vi "Populate Yokogawa Settings.vi"(4 "Sample Rate":string[](array[string]), 5 "Power  in":T2={"Yokogawa"={"WT210"={"Sample Rate (1: 0.25s)"=1, "A Range (12: 20A)"=11, "V Range (6: 600V)"=4, "Power VISA Yokogawa WT210"=""}, "WT500"={"Power VISA Yokogawa WT500"="", "V Range (8: 1000V)"=6, "I Range (7: 40A)"=7, "Update Rate (3: 500ms)"=2}}, "Aplus"={"Aplus IP Address"="192.168.1.101", "Remote Port"=502, "Instrument"="APLUS", "Instr Driver Revision"="1.03.0053"}, "Power Limits"={"Crest Factor"={"Upper Limit"=1.49, "Lower Limit"=1.34}, "Harmonic Content"={"Uthd"=2.0}, "Voltage"={"% Error"=2.0}, "Stability"={"<1 Watt "={"Wattage"=1.0, "Slope (mW/H)"=10.0}, ">1 Watt"={"1%Power/Hour"=1.0}}}, "Nominal Voltage"=120, "Time Limit (s)"=10800.0, "Power Variation Limit (%)"=50.0, "Power Supply"={"Chroma 61605"="CHROMA", "Use Chroma?"=FALSE}} {"Yokogawa"."WT500"."Update Rate (3: 500ms)" items=["-", "100ms", "200ms", "500ms", "1s", "2s", "5s"]; "Yokogawa"."WT500"."I Range (7: 40A)" items=["AUTO", "500 mA", "1 A", "2 A", "5 A", "10 A", "20 A", "40 A", "S-AUTO", "50 mV", "100 mV", "200 mV", "500 mV", "1 V", "2 V", "5 V", "10 V", "250 mA", "500 mA", "1 A", "2.5 A", "5 A", "10 A", "20 A", "25 mV", "50 mV", "100 mV", "250 mV", "500 mV", "1 V", "2.5 V", "5 V"]; "Yokogawa"."WT500"."V Range (8: 1000V)" items=["AUTO", "15", "30", "60", "100", "150", "300", "600", "1000", "7.5", "15", "30", "50", "75", "150", "300", "500"]; "Yokogawa"."WT210"."V Range (6: 600V)" items=["Auto", "15V", "30V", "60V", "150V", "300V", "600V"]; "Yokogawa"."WT210"."A Range (12: 20A)" items=["Auto", "5mA", "10mA", "20mA", "50mA", "100mA", "200mA", "0.5A", "1A", "2A", "5A", "10A", "20A", "50mV", "100mV", "200mV", "2.5V", "5V", "10V"]; "Yokogawa"."WT210"."Sample Rate (1: 0.25s)" items=["0.1s", "0.25s", "0.5s", "1s", "2s", "5s"]}, 6 "A Range":string[](array[string]), 7 "Input Array":string[][](array[string]), 8 "error in (no error)":errorcluster, 9 "V Range":string[](array[string]), 11 "Power Analyzer":T1=enum."APLUS") -> (0 "error out":errorcluster, 3 "Power  out":T2={"Yokogawa"={"WT210"={"Sample Rate (1: 0.25s)"=1, "A Range (12: 20A)"=11, "V Range (6: 600V)"=4, "Power VISA Yokogawa WT210"=""}, "WT500"={"Power VISA Yokogawa WT500"="", "V Range (8: 1000V)"=6, "I Range (7: 40A)"=7, "Update Rate (3: 500ms)"=2}}, "Aplus"={"Aplus IP Address"="192.168.1.101", "Remote Port"=502, "Instrument"="APLUS", "Instr Driver Revision"="1.03.0053"}, "Power Limits"={"Crest Factor"={"Upper Limit"=1.49, "Lower Limit"=1.34}, "Harmonic Content"={"Uthd"=2.0}, "Voltage"={"% Error"=2.0}, "Stability"={"<1 Watt "={"Wattage"=1.0, "Slope (mW/H)"=10.0}, ">1 Watt"={"1%Power/Hour"=1.0}}}, "Nominal Voltage"=120, "Time Limit (s)"=10800.0, "Power Variation Limit (%)"=50.0, "Power Supply"={"Chroma 61605"="CHROMA", "Use Chroma?"=FALSE}} {"Yokogawa"."WT500"."Update Rate (3: 500ms)" items=["-", "100ms", "200ms", "500ms", "1s", "2s", "5s"]; "Yokogawa"."WT500"."I Range (7: 40A)" items=["AUTO", "500 mA", "1 A", "2 A", "5 A", "10 A", "20 A", "40 A", "S-AUTO", "50 mV", "100 mV", "200 mV", "500 mV", "1 V", "2 V", "5 V", "10 V", "250 mA", "500 mA", "1 A", "2.5 A", "5 A", "10 A", "20 A", "25 mV", "50 mV", "100 mV", "250 mV", "500 mV", "1 V", "2.5 V", "5 V"]; "Yokogawa"."WT500"."V Range (8: 1000V)" items=["AUTO", "15", "30", "60", "100", "150", "300", "600", "1000", "7.5", "15", "30", "50", "75", "150", "300", "500"]; "Yokogawa"."WT210"."V Range (6: 600V)" items=["Auto", "15V", "30V", "60V", "150V", "300V", "600V"]; "Yokogawa"."WT210"."A Range (12: 20A)" items=["Auto", "5mA", "10mA", "20mA", "50mA", "100mA", "200mA", "0.5A", "1A", "2A", "5A", "10A", "20A", "50mV", "100mV", "200mV", "2.5V", "5V", "10V"]; "Yokogawa"."WT210"."Sample Rate (1: 0.25s)" items=["0.1s", "0.25s", "0.5s", "1s", "2s", "5s"]})   [LabVIEW 2016]
uses:
  Type Definitions/UTILITY Power Inputs Control.ctl
  Type Definitions/UTILITY Power Analyzer.ctl
  <vilib>/Instr/_visa.llb/VISA Find Search Mode.ctl
  <vilib>/Utility/error.llb/whitespace.ctl
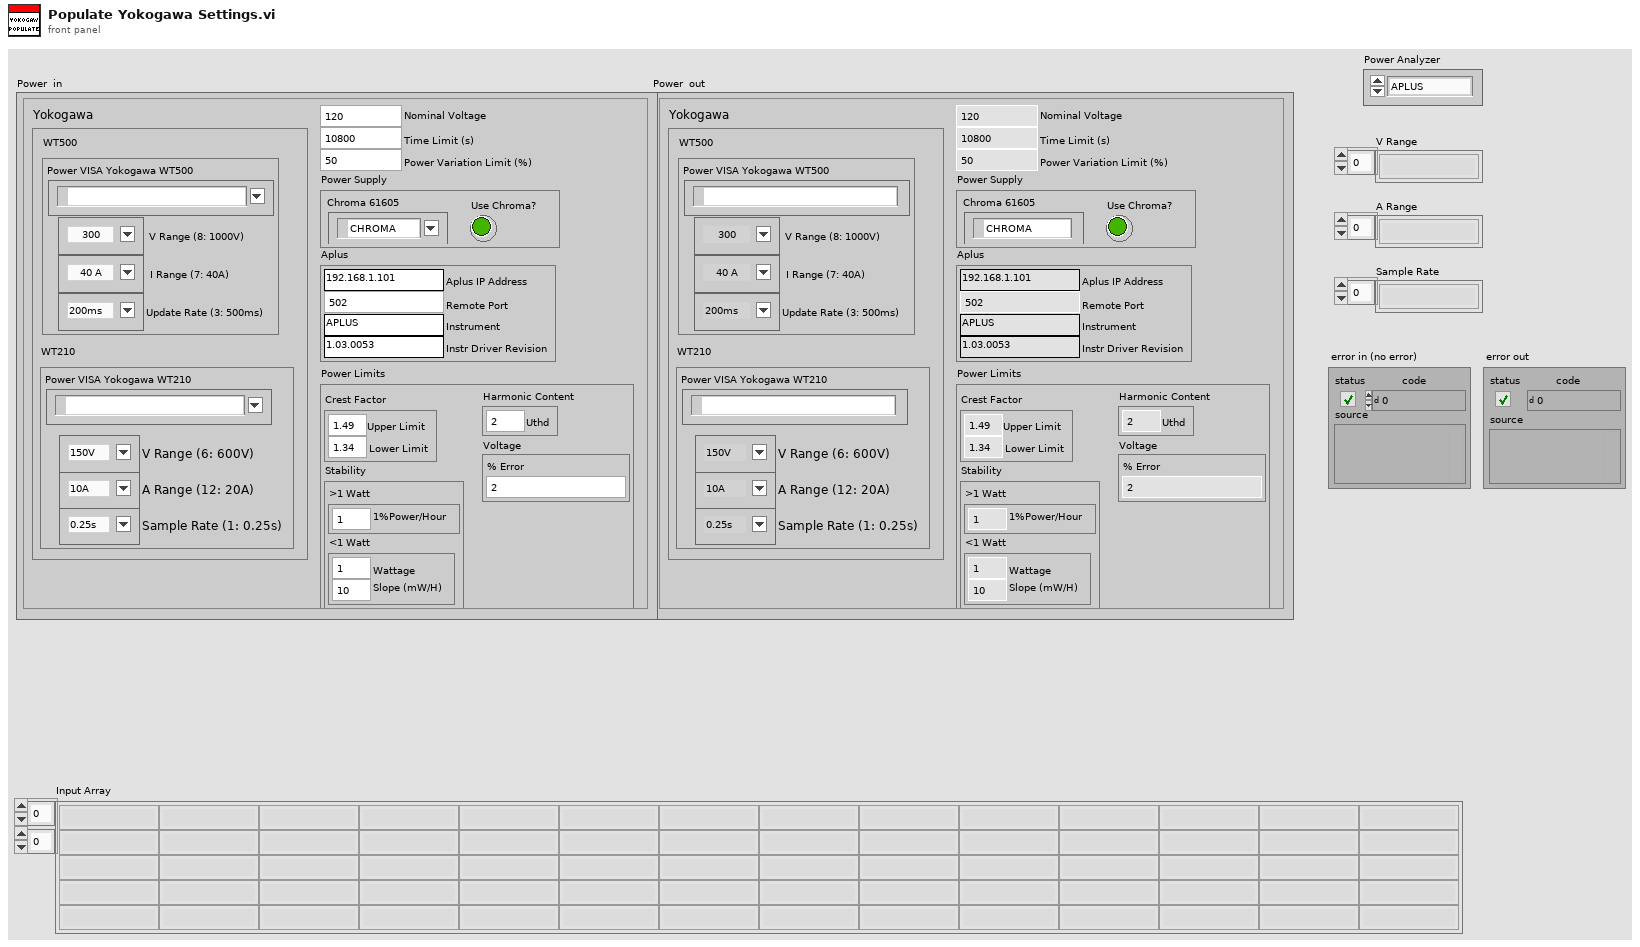
[diagram p1: front panel]
types:
  T1 = typedef "UTILITY Power Analyzer.ctl" = enum16{"", "APLUS", "WT210", "WT500", "WT300", "OSI", "Debug", "WT230"}
  T2 = typedef "UTILITY Power Inputs Control.ctl" = cluster{"Yokogawa":cluster{"WT210":cluster{"Sample Rate (1: 0.25s)":i32, "A Range (12: 20A)":i32, "V Range (6: 600V)":i32, "Power VISA Yokogawa WT210":refnum<visa-resource-name>}, "WT500":cluster{"Power VISA Yokogawa WT500":refnum<visa-resource-name>, "V Range (8: 1000V)":i32, "I Range (7: 40A)":i32, "Update Rate (3: 500ms)":i32}}, "Aplus":cluster{"Aplus IP Address":string, "Remote Port":i32, "Instrument":string, "Instr Driver Revision":string}, "Power Limits":cluster{"Crest Factor":cluster{"Upper Limit":dbl, "Lower Limit":dbl}, "Harmonic Content":cluster{"Uthd":dbl}, "Voltage":cluster{"% Error":dbl}, "Stability":cluster{"<1 Watt ":cluster{"Wattage":dbl, "Slope (mW/H)":dbl}, ">1 Watt":cluster{"1%Power/Hour":dbl}}}, "Nominal Voltage":i32, "Time Limit (s)":dbl, "Power Variation Limit (%)":dbl, "Power Supply":cluster{"Chroma 61605":refnum<visa-resource-name>, "Use Chroma?":bool}}
  T3 = typedef "VISA Find Search Mode.ctl" = u32
  T4 = typedef "whitespace.ctl" = u16
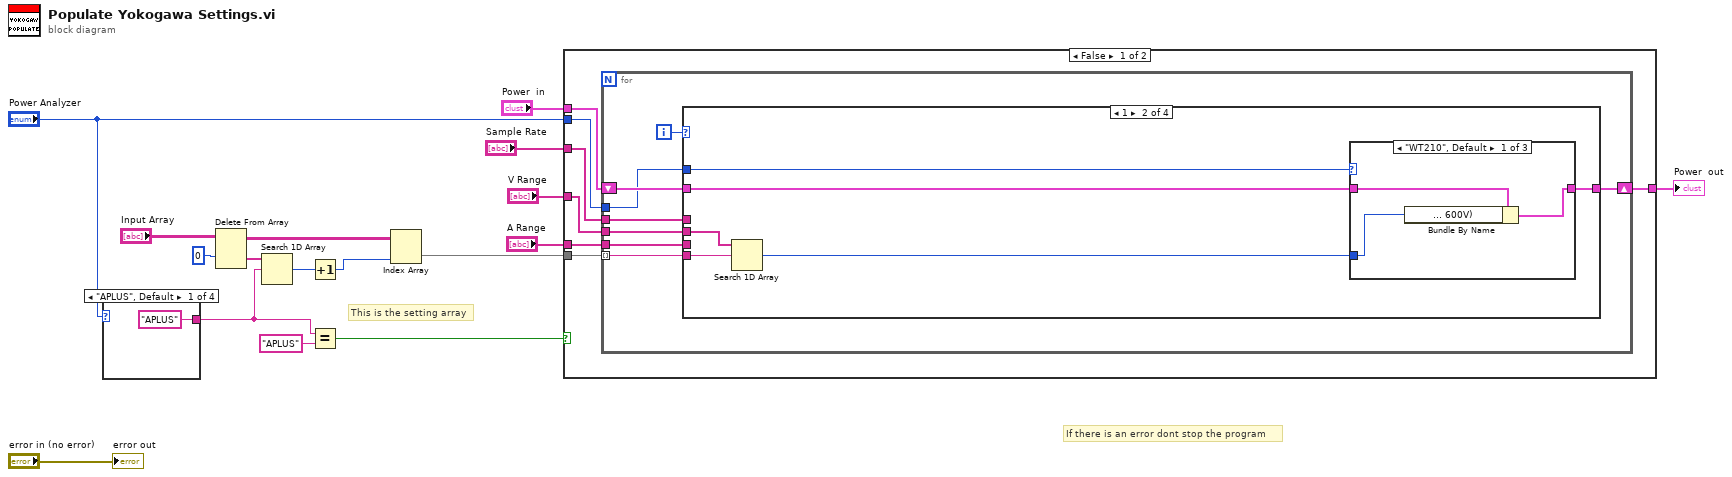
[diagram p0: block diagram]
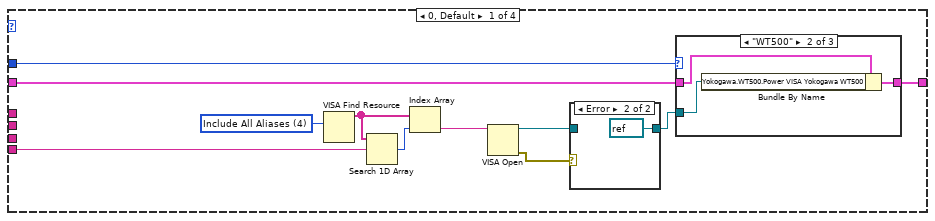
[diagram p2: hidden frame]
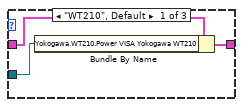
[diagram p4: hidden frame]
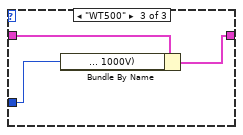
[diagram p7: hidden frame]
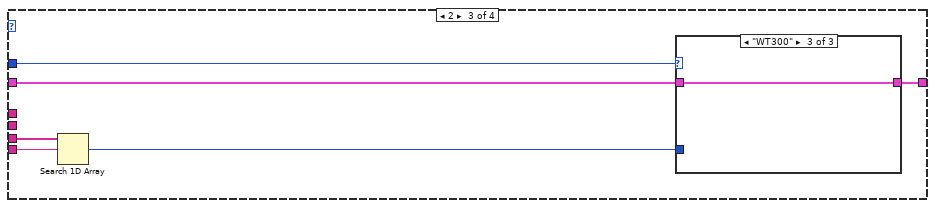
[diagram p8: hidden frame]
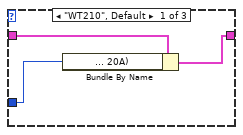
[diagram p9: hidden frame]
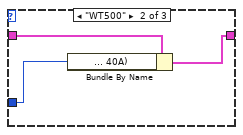
[diagram p10: hidden frame]
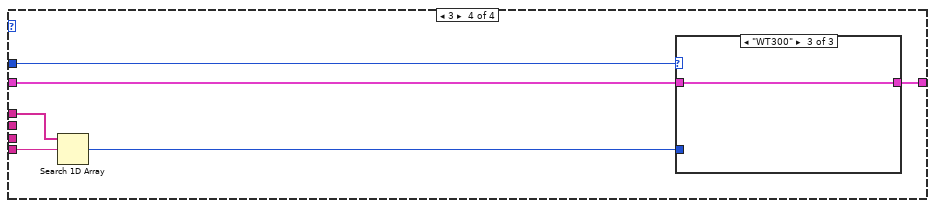
[diagram p11: hidden frame]
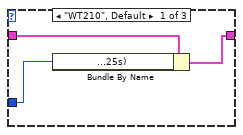
[diagram p12: hidden frame]
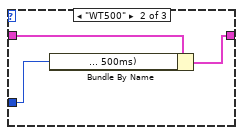
[diagram p13: hidden frame]
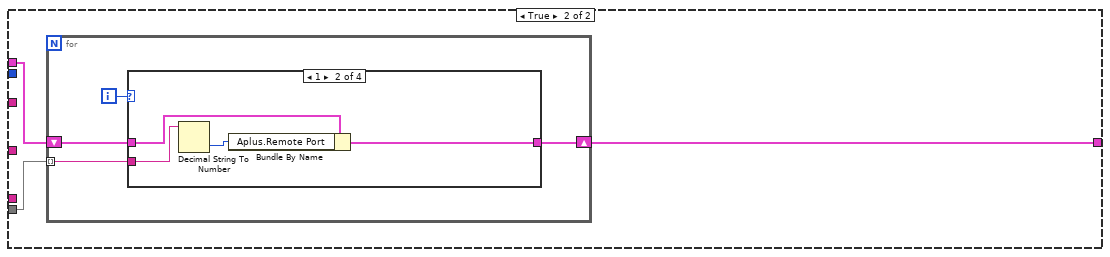
[diagram p14: hidden frame]
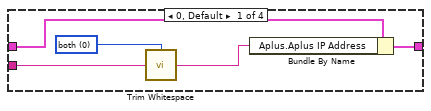
[diagram p15: hidden frame]
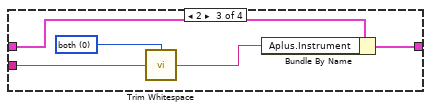
[diagram p16: hidden frame]
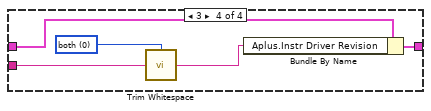
[diagram p17: hidden frame]
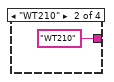
[diagram p18: hidden frame]
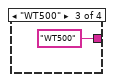
[diagram p19: hidden frame]
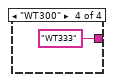
[diagram p20: hidden frame]
diagram:
  # "If there is an error dont stop the program"
  # "This is the setting array"
  n1 = case shown="\"APLUS\", Default" "Power Analyzer" {
    tunnel: ["APLUS" "WT210" "WT500" "WT333"] -> w2
    frame "APLUS", Default {
    }
    frame "WT210" {
    }
    frame "WT500" {
    }
    frame "WT300" {
    }
  }
  n2 = Delete From Array(array="Input Array", index (row)=0) -> (deleted portion=w7:string[], array with subset deleted=w8:string[][])  [unwired: 2 in]
  n3 = Search 1D Array(1D array=w7, element=w2) -> (index of element=w5:i32)  [unwired: 1 in]
  n4 = Increment(x=w5) -> (x+1=w12:i32)
  n5 = Equal?(x=w2, y="APLUS") -> (x = y?=w4:bool)
  n6 = Index Array(array=w8, index (col)=w12) -> (element=w11:string[])  [unwired: 1 in]
  n7 = case shown="False" w4 {
    tunnel: "Sample Rate" -> [w28 _]
    tunnel: "A Range" -> [w27 _]
    tunnel: "V Range" -> [w26 _]
    tunnel: [w25 w96] -> w14
    tunnel: "Power  in" -> [w24 w97]
    tunnel: w11 -> [w23 w98]
    tunnel: "Power Analyzer" -> [w22 _]
    frame False {
      n8 = for {
        tunnel: w23 -> [w34] mode=indexing
        shift-right: [w33] -> w25
        shift-left: w24 -> [w35]
        tunnel: w22 -> [w32]
        tunnel: w26 -> [w31]
        tunnel: w27 -> [w30]
        tunnel: w28 -> [w29]
        i -> [w36]
        n9 = case shown="1" w36 {
          tunnel: w35 -> [w47 w62 w75 w88]
          tunnel: [w46 w61 w74 w87] -> w33
          tunnel: w34 -> [w41 w60 w73 w86]
          tunnel: w32 -> [w40 w57 w70 w83]
          tunnel: w31 -> [_ w58 _ _]
          tunnel: w30 -> [_ _ w71 _]
          tunnel: w29 -> [_ _ _ w84]
          frame 0, Default {
            w45 = T3 4 items=["Canonical Names Only"=0, "Aliases Only"=2, "Include Matching Aliases"=3, "Include All Aliases"=4] ("Search Mode")
            n10 = VISA Find Resource(10:w45) -> (3:w43:string[])  [unwired: 2 in, 2 out]
            n11 = Search 1D Array(1D array=w43, element=w41) -> (index of element=w44:i32)  [unwired: 1 in]
            n12 = Index Array(array=w43, index=w44) -> (element=w42:string)
            n13 = VISA Open(VISA resource name=w42) -> (VISA resource name=w38:refnum<visa-resource-name>, error out=w39:errorcluster)  [unwired: 4 in]
            n14 = case shown="Error" w39 {
              tunnel: w38 -> [w48 _]
              tunnel: [w48 refnum<visa-resource-name> refnum ("VISA resource name")] -> w37
              frame No Error {
              }
              frame Error {
              }
            }
            n15 = case shown="\"WT500\"" w40 {
              tunnel: w47 -> [w52 w55 w56]
              tunnel: [w51 w54 w56] -> w46
              tunnel: w37 -> [w50 w53 _]
              frame "WT210", Default {
                n16 = Bundle By Name(cluster=w52, "Yokogawa.WT210.Power VISA Yokogawa WT210"=w50) -> (w51:T2)
              }
              frame "WT500" {
                n17 = Bundle By Name(cluster=w55, "Yokogawa.WT500.Power VISA Yokogawa WT500"=w53) -> (w54:T2)
              }
              frame "WT300" {
              }
            }
          }
          frame 1 {
            n18 = Search 1D Array(1D array=w58, element=w60) -> (index of element=w59:i32)  [unwired: 1 in]
            n19 = case shown="\"WT210\", Default" w57 {
              tunnel: w62 -> [w65 w66 w69]
              tunnel: [w64 w66 w68] -> w61
              tunnel: w59 -> [w63 _ w67]
              frame "WT210", Default {
                n20 = Bundle By Name(cluster=w65, "Yokogawa.WT210.V Range (6: 600V)"=w63) -> (w64:T2)
              }
              frame "WT300" {
              }
              frame "WT500" {
                n21 = Bundle By Name(cluster=w69, "Yokogawa.WT500.V Range (8: 1000V)"=w67) -> (w68:T2)
              }
            }
          }
          frame 2 {
            n22 = Search 1D Array(1D array=w71, element=w73) -> (index of element=w72:i32)  [unwired: 1 in]
            n23 = case shown="\"WT300\"" w70 {
              tunnel: w75 -> [w77 w81 w82]
              tunnel: [w78 w80 w82] -> w74
              tunnel: w72 -> [w76 w79 _]
              frame "WT210", Default {
                n24 = Bundle By Name(cluster=w77, "Yokogawa.WT210.A Range (12: 20A)"=w76) -> (w78:T2)
              }
              frame "WT500" {
                n25 = Bundle By Name(cluster=w81, "Yokogawa.WT500.I Range (7: 40A)"=w79) -> (w80:T2)
              }
              frame "WT300" {
              }
            }
          }
          frame 3 {
            n26 = Search 1D Array(1D array=w84, element=w86) -> (index of element=w85:i32)  [unwired: 1 in]
            n27 = case shown="\"WT300\"" w83 {
              tunnel: w88 -> [w89 w94 w95]
              tunnel: [w90 w93 w95] -> w87
              tunnel: w85 -> [w91 w92 _]
              frame "WT210", Default {
                n28 = Bundle By Name(cluster=w89, "Yokogawa.WT210.Sample Rate (1: 0.25s)"=w91) -> (w90:T2)
              }
              frame "WT500" {
                n29 = Bundle By Name(cluster=w94, "Yokogawa.WT500.Update Rate (3: 500ms)"=w92) -> (w93:T2)
              }
              frame "WT300" {
              }
            }
          }
        }
      }
    }
    frame True {
      n30 = for {
        tunnel: w98 -> [w101] mode=indexing
        shift-right: [w99] -> w96
        shift-left: w97 -> [w100]
        i -> [w102]
        n31 = case shown="1" w102 {
          tunnel: w101 -> [w104 w109 w113 w118]
          tunnel: w100 -> [w107 w111 w116 w121]
          tunnel: [w106 w110 w115 w120] -> w99
          frame 0, Default {
            w105 = T4 0 items=["both", "start of string", "end of string"] ("location (both)")
            n32 = call <vilib>:"Trim Whitespace.vi"("string"=w104, "location (both)"=w105) -> ("trimmed string"=w103:string)
            n33 = Bundle By Name(cluster=w107, "Aplus.Aplus IP Address"=w103) -> (w106:T2)
          }
          frame 1 {
            n34 = Decimal String To Number(string=w109) -> (number=w108:i32)  [unwired: 2 in, 1 out]
            n35 = Bundle By Name(cluster=w111, "Aplus.Remote Port"=w108) -> (w110:T2)
          }
          frame 2 {
            w114 = T4 0 items=["both", "start of string", "end of string"] ("location (both)")
            n36 = call <vilib>:"Trim Whitespace.vi"("string"=w113, "location (both)"=w114) -> ("trimmed string"=w112:string)
            n37 = Bundle By Name(cluster=w116, "Aplus.Instrument"=w112) -> (w115:T2)
          }
          frame 3 {
            w119 = T4 0 items=["both", "start of string", "end of string"] ("location (both)")
            n38 = call <vilib>:"Trim Whitespace.vi"("string"=w118, "location (both)"=w119) -> ("trimmed string"=w117:string)
            n39 = Bundle By Name(cluster=w121, "Aplus.Instr Driver Revision"=w117) -> (w120:T2)
          }
        }
      }
    }
  }
  "Power  out" <- w14
  "error out" <- "error in (no error)"
